vi "GetConfiguredOptions.vi"(0 "VISA resource name":refnum<visa-resource-name>, 11 "error in":errorcluster) -> (4 "VISA resource name out":refnum<visa-resource-name>, 6 "Configured Options string":string, 8 "Configured Options":i32, 10 "Configured Options binary string":string, 15 "error out":errorcluster)   [LabVIEW 2023, in "Thermotron 8800.lvlib"]
doc: "CONF\nCommand name: Send configured options\nCommand type: System status\nDescription: The 8800 sends three coded-integer bytes. These are binary-weighted bytes that\nindicate all the system options selected at the factory for the 8800. The bytes are\ndefined below:\nBit # Definition\n0 Product temperature control\n1 Humidity system\n2 Low humidity system\n3 -10degC dew point\n4 Purge\n5 Cascade refrigeration system\n6 Power Save mode\n7 Bit 7 is not used\n8 Transducers installed\n9 Check water level\n10 Go to Stop on Therm-Alarm Trip\n11 Kill TB8/9 on Refrig Trip\n12-15 Bits 12 through 15 are not used\n16 Custom chamber\n17 SE chamber\n18 System Monitor functions\n19 Go to stop mode on System Monitor trips\n20-23 Bits 20 through 23 are not used\nSyntax: CONF?\nData type: Three bytes of coded integers\nQuery example: CONF?\n8800 response: 327987 = 00000101,00000001,00110011\nbit 7 bit 6 bit 5 bit 4 bit 3 bit 2 bit 1 bit 0\n 0 0 1 1 0 0 1 1\nbit 15 bit 14 bit 13 bit 12 bit 11 bit 10 bit 9 bit 8\n 0 0 0 0 0 0 0 1\nbit 23 bit 22 bit 21 bit 20 bit 19 bit 18 bit 17 bit 16\n 0 0 0 0 0 1 0 1\n(The 8800 is configured for product temperature control, humidity, purge, and\ncascade refrigeration; refrigeration transducers are installed; the controller is\nconfigured for chamber control; and System Monitor functions are enabled.)"
uses:
  Thermotron 8800.lvlib
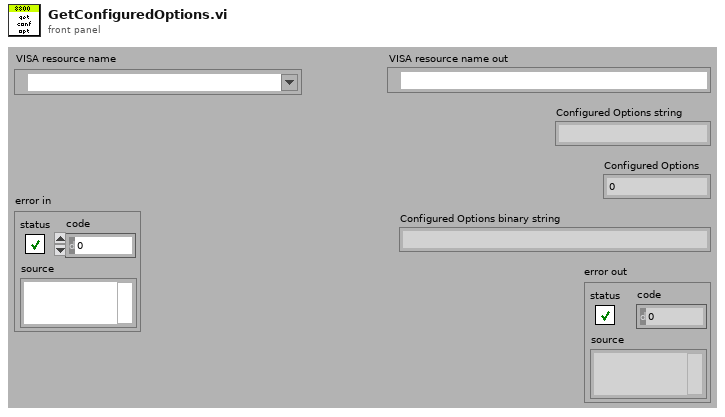
[diagram p1: front panel]
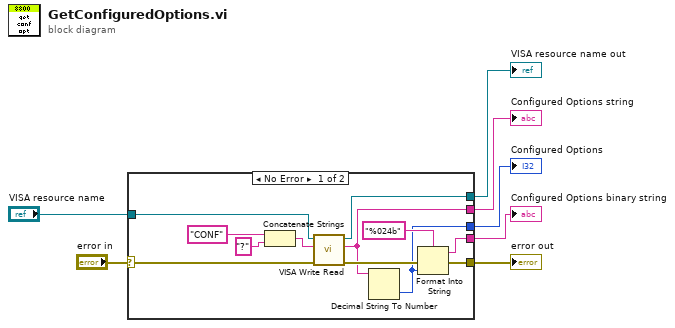
[diagram p0: block diagram]
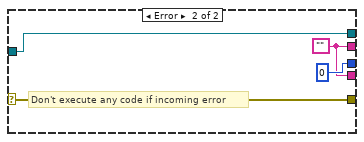
[diagram p2: hidden frame]
diagram:
  n1 = case shown="No Error" "error in" {
    selector: "error in" -> [w13 w21]
    tunnel: "VISA resource name" -> [w14 w23]
    tunnel: [w12 w21] -> w5
    tunnel: [w11 w23] -> w4
    tunnel: [w10 0] -> w3
    tunnel: [w9 w20] -> w2
    tunnel: [w8 w20] -> w1
    frame No Error {
      n2 = Concatenate Strings("CONF" ("string"), "?" ("string")) -> (w18:string)
      n3 = call "VISA Write Read.vi"("error in (no error)"=w13, "8800 Command"=w18, "VISA Refnum in"=w14) -> ("error out"=w15:errorcluster, "read buffer"=w8:string, "VISA Refnum out"=w11:refnum<visa-resource-name>)  [unwired: 6 in]
      n4 = Decimal String To Number(string=w8) -> (number=w10:i32)  [unwired: 2 in, 1 out]
      n5 = Format Into String(format string="%024b", error in=w15, w10) -> (resulting string=w9:string, error out=w12:errorcluster)  [unwired: 1 in]
    }
    frame Error {
      w20 = ""
      # "Don't execute any code if incoming error"
    }
  }
  "error out" <- w5
  "VISA resource name out" <- w4
  "Configured Options" <- w3
  "Configured Options binary string" <- w2
  "Configured Options string" <- w1
